vi "GetDiagramInputs.vi"(6 "error in":errorcluster, 9 "WhileLoop in":refnum<class "WhileLoop.lvclass">) -> (0 "error out":errorcluster, 3 "WhileLoop out":refnum<class "WhileLoop.lvclass">, 4 "inputs terminals":refnum<class "Terminal.lvclass">[][](array[class]))   [LabVIEW 2014]
uses:
  Tunnel/Tunnel.lvclass
  Terminal/Terminal.lvclass
  WhileLoop.lvclass
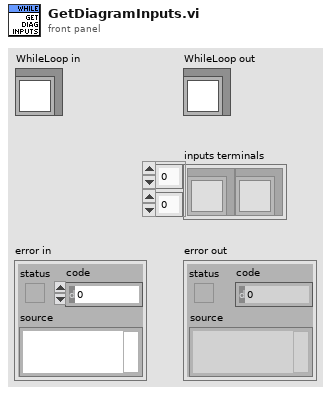
[diagram p1: front panel]
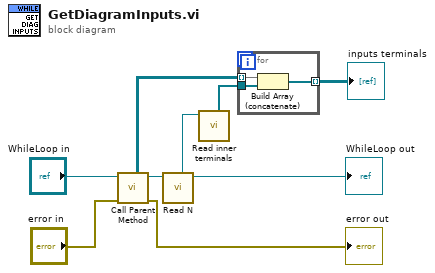
[diagram p0: block diagram]
diagram:
  n1 = call-parent "Call Parent Method"("error in"="error in", "Loop in"="WhileLoop in") -> ("error out"=→"error out":errorcluster, "Loop out"=w7:refnum<class "WhileLoop.lvclass">, "inputs terminals"=w4:refnum<class "Terminal.lvclass">[][])  [unwired: 5 in]
  n2 = call "Read N.vi"("ForLoop in"=w7) -> ("ForLoop out"=→"WhileLoop out":refnum<class "WhileLoop.lvclass">, "N"=w2:refnum<class "Tunnel.lvclass">)  [unwired: 7 in]
  n3 = call "Read inner terminals.vi"("Tunnel in"=w2) -> ("inner terminals"=w1:refnum<class "Terminal.lvclass">[])  [unwired: 7 in, 1 out]
  n4 = for {
    tunnel: w1 -> [w12]
    tunnel: w4 -> [w11] mode=indexing
    tunnel: [w10] -> w3 mode=indexing
    n5 = Build Array (concatenate)(w11, w12) -> (w10:refnum<class "Terminal.lvclass">[])
  }
  "inputs terminals" <- w3
